vi "Write message.vi"(8 "error in (no error)":errorcluster, 9 "Message type":string(combo), 10 "Message.lvclass":refnum<class "Message.lvclass">, 11 "Control-Client in":refnum<class "Control-Client.lvclass">) -> (0 "error out":errorcluster, 3 "Control-Client out":refnum<class "Control-Client.lvclass">)   [LabVIEW 2015]
uses:
  Control-Client.lvclass
  Message/Message.lvclass
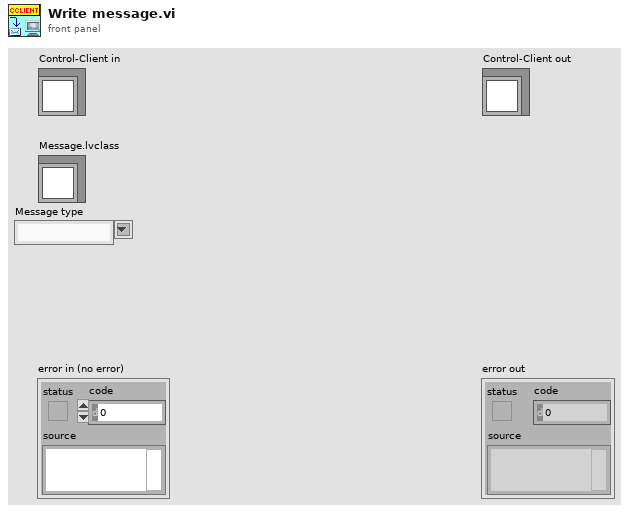
[diagram p1: front panel]
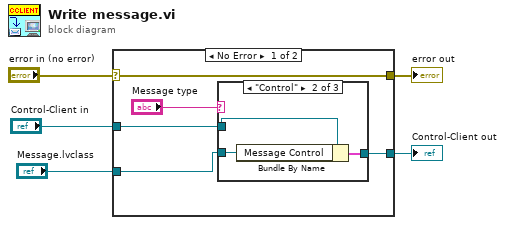
[diagram p0: block diagram]
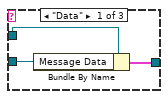
[diagram p2: hidden frame]
diagram:
  n1 = case shown="No Error" "error in (no error)" {
    selector: "error in (no error)" -> [w10 w18]
    tunnel: [w10 w18] -> w4
    tunnel: [w7 w19] -> w2
    tunnel: "Control-Client in" -> [w9 w19]
    tunnel: "Message.lvclass" -> [w8 _]
    frame No Error {
      n2 = case shown="\"Control\"" "Message type" {
        tunnel: [w11 w15 w17] -> w7
        tunnel: w9 -> [w13 w16 w17]
        tunnel: w8 -> [w12 w14 _]
        frame "Data" {
          n3 = Bundle By Name(cluster=w13, "Message Data"=w12) -> (w11:cluster{})
        }
        frame "Control" {
          n4 = Bundle By Name(cluster=w16, "Message Control"=w14) -> (w15:cluster{})
        }
        frame Default {
        }
      }
    }
    frame Error {
    }
  }
  "error out" <- w4
  "Control-Client out" <- w2
